vi "LED_test2.vi"() -> ()   [LabVIEW 2012]
uses:
  <vilib>/Utility/file.llb/Read From Spreadsheet File (DBL).vi
  <vilib>/gmath/NI_Gmath.lvlib
  <vilib>/Analysis/NI_AALPro.lvlib
panel:
  out "All Data":string[][](table)
  out "All Counts":dbl[][](array[numeric])
  out "All Abs Irr":dbl[][](array[numeric])
  out "Voltage (Lum)":dbl
  out "Voltage (Cur. Eff.)":dbl
  out "Voltage (EQE)":dbl
  out "Voltage (Lum. Pow. Eff.)":dbl
  in  "Vth_def":dbl=2.1
  out "Von":dbl
  out "Max Cur. Eff.":dbl
  out "Max Lum. Pow. Eff":dbl
  out "Max EQE":dbl
  out "Max Lum.":dbl
  out "Counts/Abs. Irr. vs Wavelength":cluster{"Y":dbl[], "Y":dbl[]}[](graph)
  out "Cur. Eff./Lum. Pow. Eff. vs Voltage":cluster{"Y":dbl[], "Y":dbl[]}[](graph)
  out "Lum. Pow. Eff vs Lum./Cur. Den.":cluster{"Y":dbl[], "Y":dbl[]}[](graph)
  out "Cur. Den. /Lum. vs Voltage":cluster{"Y":dbl[], "Y":dbl[]}[](graph)
  out "Cur. Eff. vs Lum./Cur. Den.":cluster{"Y":dbl[], "Y":dbl[]}[](graph)
  out "x2":dbl=3e-06
  out "x1":dbl=3e-06
  out "WL_1":dbl
  out "WL_2":dbl
  in  "WL_high":dbl=1131.0
  in  "WL_low":dbl=348.0
  out "EQE_array":dbl[](array[numeric])
  out "EQE vs Lum./Cur. Den.":T1(graph)
  out "XY Graph 3":cluster{"Wavelength":dbl[], "Counts":dbl[]}(graph)
  out "Luminance Ratio":dbl[](array[numeric])
  out "Calculated_luminance_array":dbl[](array[numeric])
  out "Calculated_candela_array":dbl[](array[numeric])
  out "Photon_count_array":dbl[](array[numeric])
  out "Photon_count":dbl
  out "Energy_WL":dbl[](array[numeric])
  out "Calculated_candela":dbl
  out "Abs_irr_itpl":dbl[](array[numeric]) format="%_6g"
  out "WL itpl 2":dbl[](array[numeric]) format="%_6g"
  out "Luminous Power Efficiency":dbl[](array[numeric])
  out "current efficiency (Cd/A)":dbl[](array[numeric])
  out "current density (mA/cm2)":dbl[](array[numeric])
  in  "Device Area (m2)":dbl=3e-06
  out "WL_spectrum":dbl[](array[numeric])
  out "Counts_spectrum":dbl[](array[numeric])
  out "Abs_Irr_spectrum":dbl[](array[numeric])
  out "Spectrum":dbl[][](array[numeric])
  out "Counts_dark_spectrum":dbl[](array[numeric])
  out "WL_dark_spectrum":dbl[](array[numeric])
  out "Dark Spectrum all":dbl[][](array[numeric]) format="%0.3f"
  out "Dark_spectrum":dbl[][](array[numeric])
  out "All Spectrum":dbl[][](array[numeric])
  in  "Spectrum File":path=path "W:/LED_quickVIEW/For calibration/20170914_194634spectrum_raw.ciemo"
  out "uW":dbl[](array[numeric])
  out "Luminance":dbl[](array[numeric])
  out "Candela":dbl[](array[numeric])
  out "Current":dbl[](array[numeric])
  out "Voltage":dbl[](array[numeric])
  out "Data":dbl[][](array[numeric]) format="%#.3e"
  in  "Data File":path=path "W:/LED_quickVIEW/For calibration/20170914_194634data.ciemo"
  in  "Calibration File":path=path "W:/LED_quickVIEW/For calibration/2016-12-19 callibration_OOIIrrad.cal_OOIIrrad.cal_OOIIrrad.cal"
  in  "Dark Spectrum File":path=path "W:/LED_quickVIEW/For calibration/20170914_194634dark_reference.ciemo"
  out "max value":dbl
  out "Peak Position":dbl
  out "max index(es)":i32
  out "Iso. Coef. itpl":dbl[](array[numeric]) format="%_6g"
  out "WL itpl":dbl[](array[numeric]) format="%_6g"
  out "XY Graph 2":cluster{"WL":dbl[], "Iso. Coef.":dbl[]}[](graph)
  out "Iso. Coef.":dbl[](array[numeric])
  out "WL":dbl[](array[numeric])
  out "Wavelength":dbl[](array[numeric])
  out "Counts to Abs Irr":dbl[](array[numeric])
  out "XY Graph":cluster{"Wavelength":dbl[], "Counts":dbl[]}(graph)
  out "subarray":dbl[][](array[numeric])
  out "array":dbl[][](array[numeric])
  # "From"
  # "To"
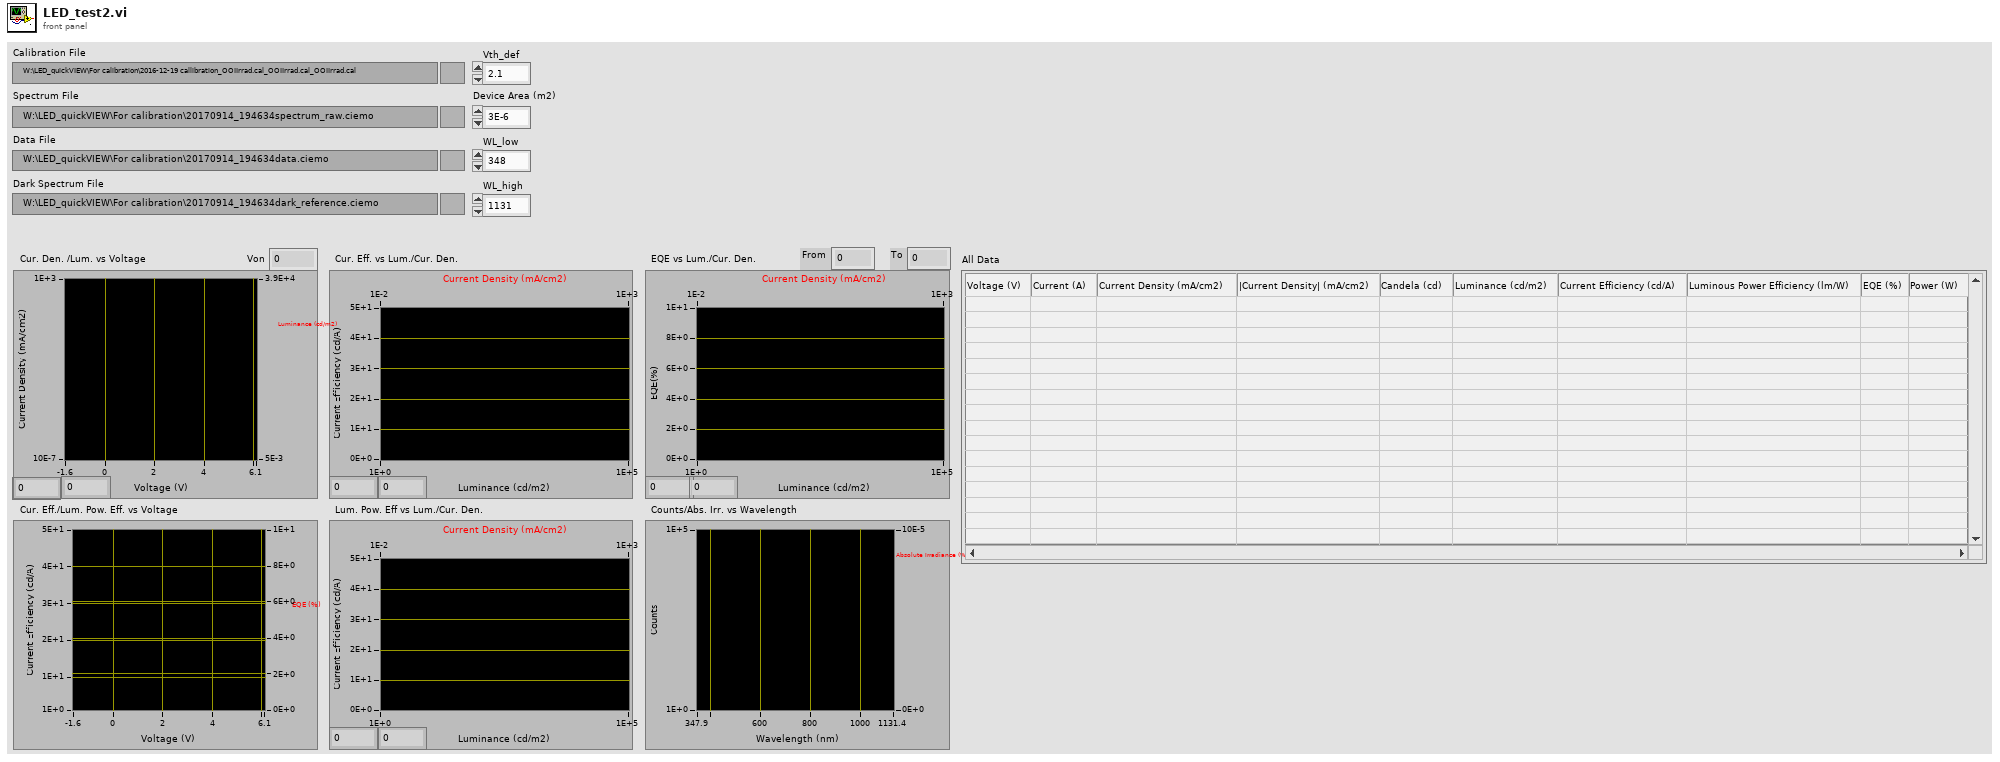
[diagram p1: front panel]
types:
  T1 = cluster{"current density (mA/cm2)":dbl[], "EQE_array":dbl[]}[]
  T2 = cluster{"Wavelength":dbl[], "Counts to Abs Irr":dbl[]}
  T3 = cluster{"WL itpl":dbl[], "Iso. Coef. itpl":dbl[]}
  T4 = cluster{"WL itpl":dbl[], "Iso. Coef. itpl":dbl[]}[]
  T5 = cluster{"Luminance":dbl[], "current efficiency (Cd/A)":dbl[]}
  T6 = cluster{"current density (mA/cm2)":dbl[], "current efficiency (Cd/A)":dbl[]}
  T7 = cluster{"current density (mA/cm2)":dbl[], "EQE_array":dbl[]}
  T8 = cluster{"current density (mA/cm2)":dbl[], "current efficiency (Cd/A)":dbl[]}[]
  T9 = cluster{"Voltage":dbl[], "current efficiency (Cd/A)":dbl[]}
  T10 = cluster{"Luminance":dbl[], "Luminous Power Efficiency":dbl[]}
  T11 = cluster{"current density (mA/cm2)":dbl[], "Luminous Power Efficiency":dbl[]}
  T12 = cluster{"current density (mA/cm2)":dbl[], "Luminous Power Efficiency":dbl[]}[]
  T13 = cluster{"WL_spectrum":dbl[], "Counts_spectrum":dbl[]}
  T14 = cluster{"WL_spectrum":dbl[], "Abs_Irr_spectrum":dbl[]}
  T15 = cluster{"WL_spectrum":dbl[], "Abs_Irr_spectrum":dbl[]}[]
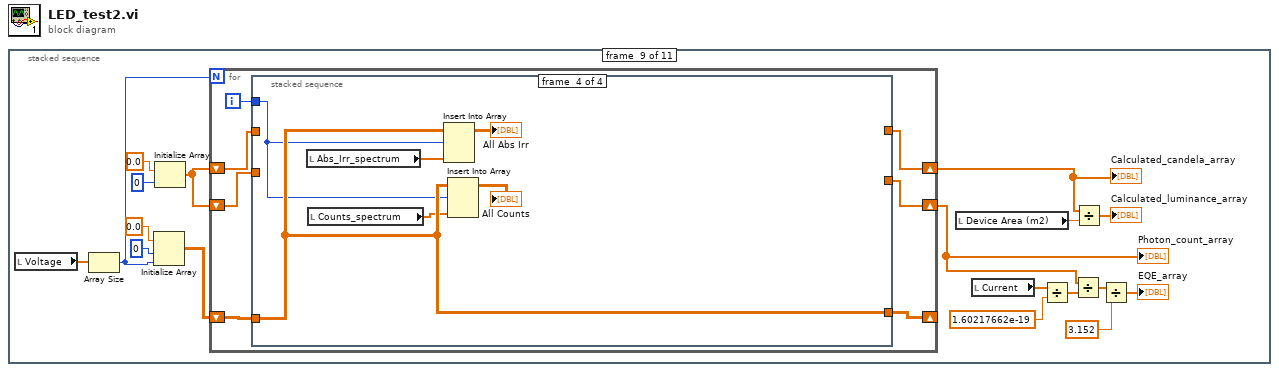
[diagram p0: block diagram]
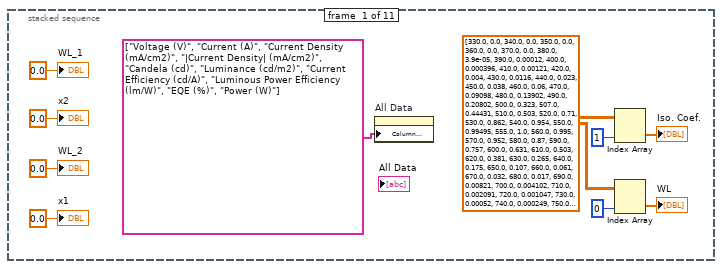
[diagram p2: hidden frame]
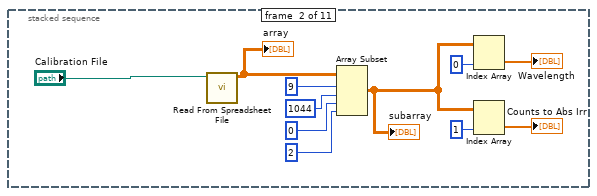
[diagram p3: hidden frame]
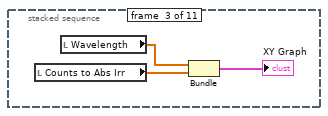
[diagram p4: hidden frame]
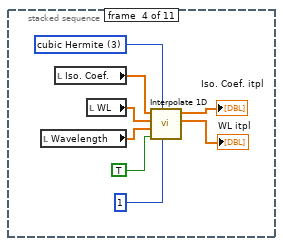
[diagram p5: hidden frame]
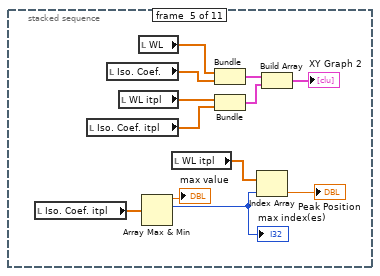
[diagram p6: hidden frame]
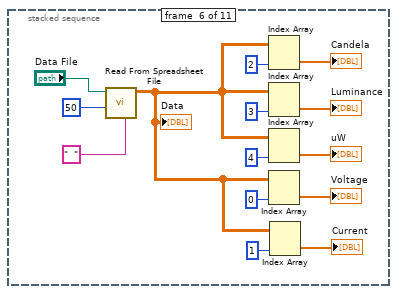
[diagram p7: hidden frame]
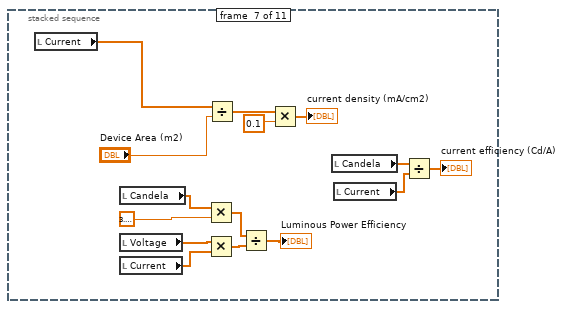
[diagram p8: hidden frame]
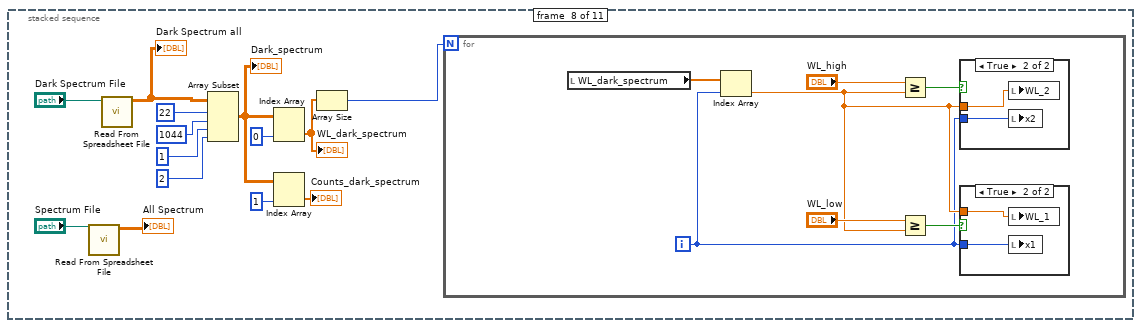
[diagram p9: hidden frame]
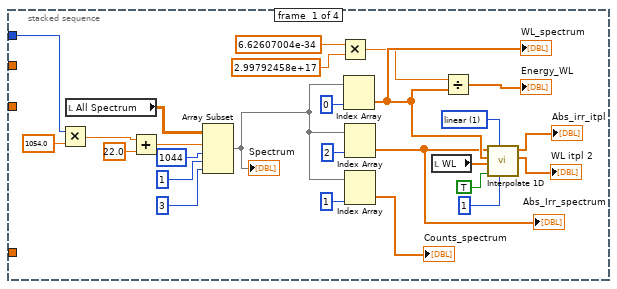
[diagram p12: hidden frame]
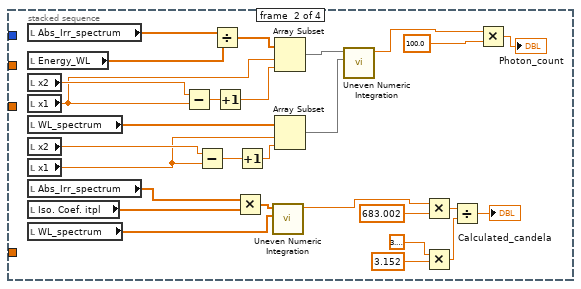
[diagram p13: hidden frame]
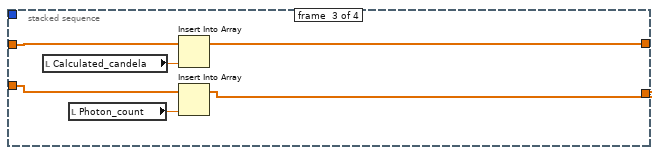
[diagram p14: hidden frame]
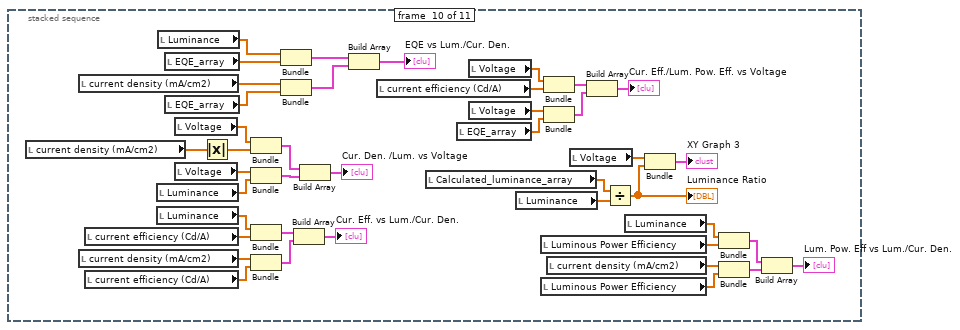
[diagram p15: hidden frame]
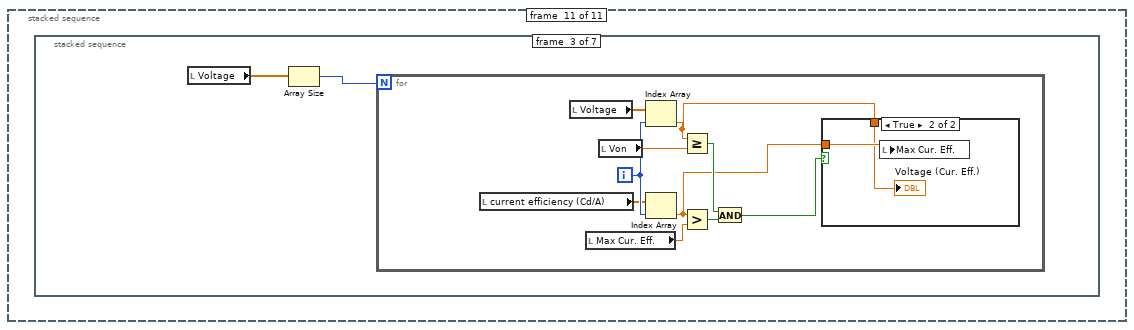
[diagram p16: hidden frame]
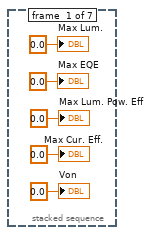
[diagram p17: hidden frame]
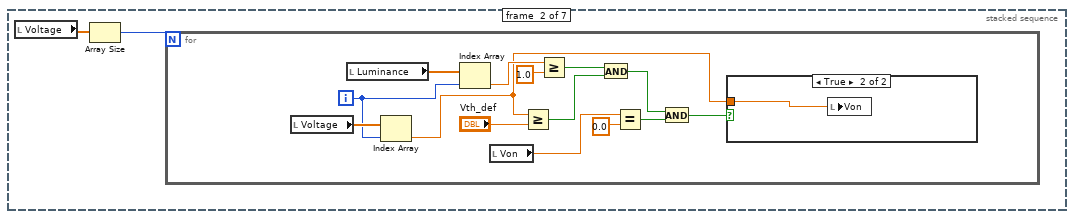
[diagram p18: hidden frame]
diagram:
  n1 = stacked-sequence {
    frame #0 {
      w9 = dbl[][] [[330.0, 0.0], [340.0, 0.0], [350.0, 0.0], [360.0, 0.0], [370.0, 0.0], [380.0, 3.9e-05], [390.0, 0.00012], [400.0, 0.000396], [410.0, 0.00121], [420.0, 0.004], [430.0, 0.0116], [440.0, 0.023], [450.0, 0.038], [460.0, 0.06], [470.0, 0.09098], [480.0, 0.13902], [490.0, 0.20802], [500.0, 0.323], [507.0, 0.44431], [510.0, 0.503], [520.0, 0.71], [530.0, 0.862], [540.0, 0.954], [550.0, 0.99495], [555.0, 1.0], [560.0, 0.995], [570.0, 0.952], [580.0, 0.87], [590.0, 0.757], [600.0, 0.631], [610.0, 0.503], [620.0, 0.381], [630.0, 0.265], [640.0, 0.175], [650.0, 0.107], [660.0, 0.061], [670.0, 0.032], [680.0, 0.017], [690.0, 0.00821], [700.0, 0.004102], [710.0, 0.002091], [720.0, 0.001047], [730.0, 0.00052], [740.0, 0.000249], [750.0, 0.00012], [760.0, 6e-05], [770.0, 3e-05], [780.0, 0.0], [790.0, 0.0], [800.0, 0.0], [810.0, 0.0], [820.0, 0.0], [830.0, 0.0], [840.0, 0.0], [850.0, 0.0], [860.0, 0.0], [870.0, 0.0], [880.0, 0.0], [890.0, 0.0], [900.0, 0.0], [910.0, 0.0], [920.0, 0.0], [930.0, 0.0], [940.0, 0.0], [950.0, 0.0], [960.0, 0.0], [970.0, 0.0], [980.0, 0.0], [990.0, 0.0], [1000.0, 0.0], [1010.0, 0.0], [1020.0, 0.0], [1030.0, 0.0], [1040.0, 0.0], [1050.0, 0.0], [1060.0, 0.0], [1070.0, 0.0], [1080.0, 0.0], [1090.0, 0.0], [1100.0, 0.0], [1110.0, 0.0], [1120.0, 0.0], [1130.0, 0.0], [1140.0, 0.0]] ("all rows")
      n2 = property on="All Data" class="Tbl (strict)"("Column Headers[]"=string[] ["Voltage (V)", "Current (A)", "Current Density (mA/cm2)", "|Current Density| (mA/cm2)", "Candela (cd)", "Luminance (cd/m2)", "Current Efficiency (cd/A)", "Luminous Power Efficiency (lm/W)", "EQE (%)", "Power (W)"] ("Row Header Strings[]")) -> ()  [unwired: 2 in, 2 out]
      n3 = Index Array(array=w9, index (col)=1 ("disabled index (col)")) -> (element=→"Iso. Coef.":dbl[])  [unwired: 1 in]
      n4 = Index Array(array=w9, index (col)=0 ("disabled index (col)")) -> (element=→"WL":dbl[])  [unwired: 1 in]
      "WL_2" <- 0.0 ("WL_2")
      "WL_1" <- 0.0 ("WL_1")
      "x1" <- 0.0 ("x1")
      "x2" <- 0.0 ("x2")
    }
    frame #1 {
      n5 = call-poly <vilib>:"Read From Spreadsheet File.vi"("file path (dialog if empty)"="Calibration File") -> ("all rows"=w18:dbl[][])  [unwired: 6 in, 4 out]
      "array" <- w18
      n6 = Array Subset(array=w18, index (row)=9 ("index"), length (row)=1044 ("length"), index (col)=0 ("index"), length (col)=2 ("length")) -> (w15:dbl[][])
      "subarray" <- w15
      n7 = Index Array(array=w15, index (col)=0 ("index")) -> (element=→"Wavelength":dbl[])  [unwired: 1 in]
      n8 = Index Array(array=w15, index (col)=1 ("length")) -> (element=→"Counts to Abs Irr":dbl[])  [unwired: 1 in]
    }
    frame #2 {
      n9 = local read "Counts to Abs Irr"() -> (w22:dbl[])
      n10 = local read "Wavelength"() -> (w23:dbl[])
      n11 = Bundle("Wavelength"=w23, "Counts to Abs Irr"=w22) -> (→"XY Graph":T2)  [unwired: 1 in]
    }
    frame #3 {
      w28 = 3 items=["nearest", "linear", "spline", "cubic Hermite", "Lagrange"] ("method")
      n12 = local read "Wavelength"() -> (w30:dbl[])
      n13 = local read "Iso. Coef."() -> (w31:dbl[])
      n14 = local read "WL"() -> (w32:dbl[])
      n15 = call <vilib>:"Interpolate 1D.vi"("ntimes"=1, "method"=w28, "X is monotonic"=TRUE, "xi"=w30, "X"=w32, "Y"=w31) -> ("xi used"=→"WL itpl":dbl[], "yi"=→"Iso. Coef. itpl":dbl[])  [unwired: 3 in, 1 out]
    }
    frame #4 {
      n16 = local read "Iso. Coef. itpl"() -> (w37:dbl[])
      n17 = local read "Iso. Coef. itpl"() -> (w33:dbl[])
      n18 = local read "Iso. Coef."() -> (w44:dbl[])
      n19 = local read "WL itpl"() -> (w41:dbl[])
      n20 = local read "WL"() -> (w43:dbl[])
      n21 = Array Max & Min(array=w37) -> (max value=→"max value":dbl, max index (indices)=w40:i32)  [unwired: 2 out]
      "max index(es)" <- w40
      n22 = local read "WL itpl"() -> (w39:dbl[])
      n23 = Bundle("WL"=w43, "Iso. Coef."=w44) -> (w42:cluster{"WL":dbl[], "Iso. Coef.":dbl[]})  [unwired: 1 in]
      n24 = Bundle("WL itpl"=w41, "Iso. Coef. itpl"=w33) -> (w34:T3)  [unwired: 1 in]
      n25 = Index Array(array=w39, index=w40) -> (element=→"Peak Position":dbl)
      n26 = Build Array(w42, w34) -> (→"XY Graph 2":T4)
    }
    frame #5 {
      n27 = call-poly <vilib>:"Read From Spreadsheet File.vi"("delimiter (\\t)"="  " ("delimiter (\\t)"), "start of read offset (chars.:0)"=50, "file path (dialog if empty)"="Data File") -> ("all rows"=w46:dbl[][])  [unwired: 4 in, 4 out]
      "Data" <- w46
      n28 = Index Array(array=w46, index (col)=2 ("index (row)")) -> (element=→"Candela":dbl[])  [unwired: 1 in]
      n29 = Index Array(array=w46, index (col)=3 ("index (row)")) -> (element=→"Luminance":dbl[])  [unwired: 1 in]
      n30 = Index Array(array=w46, index (col)=4 ("index (row)")) -> (element=→"uW":dbl[])  [unwired: 1 in]
      n31 = Index Array(array=w46, index (col)=0 ("index (row)")) -> (element=→"Voltage":dbl[])  [unwired: 1 in]
      n32 = Index Array(array=w46, index (col)=1 ("index (row)")) -> (element=→"Current":dbl[])  [unwired: 1 in]
    }
    frame #6 {
      n33 = local read "Current"() -> (w66:dbl[])
      n34 = local read "Candela"() -> (w61:dbl[])
      n35 = local read "Voltage"() -> (w63:dbl[])
      n36 = local read "Current"() -> (w62:dbl[])
      n37 = Multiply(x=w61, y=3.141592653589793) -> (x*y=w64:dbl[])
      n38 = Multiply(x=w63, y=w62) -> (x*y=w65:dbl[])
      n39 = Divide(x=w66, y="Device Area (m2)") -> (x/y=w71:dbl[])
      n40 = Divide(x=w64, y=w65) -> (x/y=→"Luminous Power Efficiency":dbl[])
      n41 = Multiply(x=w71, y=0.1) -> (x*y=→"current density (mA/cm2)":dbl[])
      n42 = local read "Candela"() -> (w68:dbl[])
      n43 = local read "Current"() -> (w69:dbl[])
      n44 = Divide(x=w68, y=w69) -> (x/y=→"current efficiency (Cd/A)":dbl[])
    }
    frame #7 {
      n45 = call-poly <vilib>:"Read From Spreadsheet File.vi"("file path (dialog if empty)"="Spectrum File") -> ("all rows"=→"All Spectrum":dbl[][])  [unwired: 6 in, 4 out]
      n46 = call-poly <vilib>:"Read From Spreadsheet File.vi"("file path (dialog if empty)"="Dark Spectrum File") -> ("all rows"=w84:dbl[][])  [unwired: 6 in, 4 out]
      "Dark Spectrum all" <- w84
      n47 = Array Subset(array=w84, index (row)=22 ("index"), length (row)=1044 ("length"), index (col)=1 ("index"), length (col)=2 ("length")) -> (w76:dbl[][])
      "Dark_spectrum" <- w76
      n48 = Index Array(array=w76, index (col)=0 ("index")) -> (element=w75:dbl[])  [unwired: 1 in]
      "WL_dark_spectrum" <- w75
      n49 = Index Array(array=w76, index (col)=1 ("index")) -> (element=→"Counts_dark_spectrum":dbl[])  [unwired: 1 in]
      n50 = Array Size(array=w75) -> (size(s)=w74:i32)
      n51 = for {
        N: w74 -> [_]
        i -> [w88]
        n52 = local read "WL_dark_spectrum"() -> (w90:dbl[])
        n53 = Index Array(array=w90, index=w88) -> (element=w89:dbl)
        n54 = Greater Or Equal?(x="WL_high", y=w89) -> (x >= y?=w92:bool)
        n55 = Greater Or Equal?(x="WL_low", y=w89) -> (x >= y?=w91:bool)
        n56 = case shown="True" w92 {
          tunnel: w89 -> [_ w98]
          tunnel: w88 -> [_ w97]
          frame False {
          }
          frame True {
            n57 = local write "WL_2"(w98) -> ()
            n58 = local write "x2"(w97) -> ()
          }
        }
        n59 = case shown="True" w91 {
          tunnel: w89 -> [_ w96]
          tunnel: w88 -> [_ w95]
          frame False {
          }
          frame True {
            n60 = local write "WL_1"(w96) -> ()
            n61 = local write "x1"(w95) -> ()
          }
        }
      }
    }
    frame #8 {
      n62 = local read "Voltage"() -> (w116:dbl[])
      n63 = Array Size(array=w116) -> (size(s)=w101:i32)
      n64 = Initialize Array(0.0 ("element"), 0 ("dimension size"), w101) -> (w99:dbl[][])
      n65 = Initialize Array(0.0 ("element"), 0 ("dimension size")) -> (w103:dbl[])
      n66 = for {
        N: w101 -> [_]
        shift-right: [w121] -> w113
        shift-left: w103 -> [w122]
        shift-right: [w119] -> w108
        shift-left: w103 -> [w120]
        shift-right: [w117] -> _
        shift-left: w99 -> [w118]
        i -> [w123]
        n67 = stacked-sequence {
          tunnel: w123 -> [w137 _ _ w185]
          tunnel: w122 -> [_ _ w182 _]
          tunnel: [_ _ w181 _] -> w121
          tunnel: w120 -> [_ _ w179 _]
          tunnel: [_ _ w178 _] -> w119
          tunnel: w118 -> [_ _ _ w188]
          tunnel: [_ _ _ w188] -> w117
          frame #0 {
            w134 = 1 items=["nearest", "linear", "spline", "cubic Hermite", "Lagrange"] ("method")
            n68 = Multiply(x=w137, y=1054.0) -> (x*y=w147:dbl)
            n69 = local read "All Spectrum"() -> (w136:dbl[][])
            n70 = Add(x=w147, y=22.0) -> (x+y=w149:dbl)
            n71 = Array Subset(array=w136, index (row)=w149, length (row)=1044 ("length"), index (col)=1 ("index"), length (col)=3 ("length")) -> (w140:dbl[][])
            "Spectrum" <- w140
            n72 = Multiply(x=6.62607004e-34, y=2.99792458e+17) -> (x*y=w127:dbl)
            n73 = Index Array(array=w140, index (col)=0 ("index")) -> (element=w131:dbl[])  [unwired: 1 in]
            "WL_spectrum" <- w131
            n74 = Index Array(array=w140, index (col)=2 ("index")) -> (element=w130:dbl[])  [unwired: 1 in]
            "Abs_Irr_spectrum" <- w130
            n75 = Index Array(array=w140, index (col)=1 ("length")) -> (element=→"Counts_spectrum":dbl[])  [unwired: 1 in]
            n76 = local read "WL"() -> (w129:dbl[])
            n77 = Divide(x=w127, y=w131) -> (x/y=→"Energy_WL":dbl[])
            n78 = call <vilib>:"Interpolate 1D.vi"("ntimes"=1, "method"=w134, "X is monotonic"=TRUE, "xi"=w129, "X"=w131, "Y"=w130) -> ("xi used"=→"WL itpl 2":dbl[], "yi"=→"Abs_irr_itpl":dbl[])  [unwired: 3 in, 1 out]
          }
          frame #1 {
            n79 = local read "Abs_Irr_spectrum"() -> (w169:dbl[])
            n80 = local read "Energy_WL"() -> (w168:dbl[])
            n81 = local read "x2"() -> (w155:dbl)
            n82 = local read "x1"() -> (w154:dbl)
            n83 = local read "WL_spectrum"() -> (w151:dbl[])
            n84 = local read "x2"() -> (w153:dbl)
            n85 = local read "x1"() -> (w152:dbl)
            n86 = local read "Abs_Irr_spectrum"() -> (w177:dbl[])
            n87 = local read "Iso. Coef. itpl"() -> (w176:dbl[])
            n88 = local read "WL_spectrum"() -> (w174:dbl[])
            n89 = Subtract(x=w155, y=w154) -> (x-y=w160:dbl)
            n90 = Subtract(x=w153, y=w152) -> (x-y=w157:dbl)
            n91 = Divide(x=w169, y=w168) -> (x/y=w161:dbl[])
            n92 = Increment(x=w160) -> (x+1=w159:dbl)
            n93 = Multiply(x=w177, y=w176) -> (x*y=w175:dbl[])
            n94 = Increment(x=w157) -> (x+1=w156:dbl)
            n95 = call <vilib>:"Uneven Numeric Integration.vi"("T"=w174, "X"=w175) -> ("result"=w172:dbl)  [unwired: 8 in, 1 out]
            n96 = Array Subset(array=w161, index=w154, length=w159) -> (w158:dbl[])
            n97 = Array Subset(array=w151, index=w152, length=w156) -> (w150:dbl[])
            n98 = call <vilib>:"Uneven Numeric Integration.vi"("T"=w150, "X"=w158) -> ("result"=w167:dbl)  [unwired: 8 in, 1 out]
            n99 = Multiply(x=w172, y=683.002) -> (x*y=w173:dbl)
            n100 = Multiply(x=3.141592653589793, y=3.152) -> (x*y=w163:dbl)
            n101 = Divide(x=w173, y=w163) -> (x/y=→"Calculated_candela":dbl)
            n102 = Multiply(x=w167, y=100.0) -> (x*y=→"Photon_count":dbl)
          }
          frame #2 {
            n103 = local read "Calculated_candela"() -> (w183:dbl)
            n104 = local read "Photon_count"() -> (w180:dbl)
            n105 = Insert Into Array(array=w182, new element=w183) -> (w181:dbl[])  [unwired: 1 in]
            n106 = Insert Into Array(array=w179, new element=w180) -> (w178:dbl[])  [unwired: 1 in]
          }
          frame #3 {
            n107 = local read "Abs_Irr_spectrum"() -> (w189:dbl[])
            n108 = local read "Counts_spectrum"() -> (w187:dbl[])
            n109 = Insert Into Array(array=w188, index (row)=w185, new element=w189) -> (→"All Abs Irr":dbl[][])  [unwired: 1 in]
            n110 = Insert Into Array(array=w188, index (row)=w185, new element=w187) -> (→"All Counts":dbl[][])  [unwired: 1 in]
          }
        }
      }
      "Photon_count_array" <- w108
      "Calculated_candela_array" <- w113
      n111 = local read "Device Area (m2)"() -> (w111:dbl)
      n112 = local read "Current"() -> (w110:dbl[])
      n113 = Divide(x=w110, y=1.60217662e-19) -> (x/y=w109:dbl[])
      n114 = Divide(x=w108, y=w109) -> (x/y=w106:dbl[])
      n115 = Divide(x=w113, y=w111) -> (x/y=→"Calculated_luminance_array":dbl[])
      n116 = Divide(x=w106, y=3.152) -> (x/y=→"EQE_array":dbl[])
    }
    frame #9 {
      n117 = local read "current density (mA/cm2)"() -> (w212:dbl[])
      n118 = local read "current density (mA/cm2)"() -> (w222:dbl[])
      n119 = local read "current density (mA/cm2)"() -> (w205:dbl[])
      n120 = local read "current efficiency (Cd/A)"() -> (w207:dbl[])
      n121 = local read "current efficiency (Cd/A)"() -> (w204:dbl[])
      n122 = local read "Luminance"() -> (w213:dbl[])
      n123 = local read "Luminance"() -> (w206:dbl[])
      n124 = local read "Luminance"() -> (w223:dbl[])
      n125 = local read "EQE_array"() -> (w224:dbl[])
      n126 = local read "EQE_array"() -> (w225:dbl[])
      n127 = local read "Voltage"() -> (w215:dbl[])
      n128 = local read "Voltage"() -> (w214:dbl[])
      n129 = Absolute Value(x=w212) -> (abs(x)=w211:dbl[])
      n130 = Bundle("Voltage"=w215, w211) -> (w218:cluster{"Voltage":dbl[], dbl[]})  [unwired: 1 in]
      n131 = Bundle("Voltage"=w214, "Luminance"=w213) -> (w217:cluster{"Voltage":dbl[], "Luminance":dbl[]})  [unwired: 1 in]
      n132 = Bundle("Luminance"=w206, "current efficiency (Cd/A)"=w207) -> (w210:T5)  [unwired: 1 in]
      n133 = Bundle("current density (mA/cm2)"=w205, "current efficiency (Cd/A)"=w204) -> (w209:T6)  [unwired: 1 in]
      n134 = Bundle("Luminance"=w223, "EQE_array"=w224) -> (w221:cluster{"Luminance":dbl[], "EQE_array":dbl[]})  [unwired: 1 in]
      n135 = Bundle("current density (mA/cm2)"=w222, "EQE_array"=w225) -> (w220:T7)  [unwired: 1 in]
      n136 = Build Array(w210, w209) -> (→"Cur. Eff. vs Lum./Cur. Den.":T8)
      n137 = Build Array(w218, w217) -> (→"Cur. Den. /Lum. vs Voltage":cluster{"Voltage":dbl[], "Luminance":dbl[]}[])
      n138 = Build Array(w221, w220) -> (→"EQE vs Lum./Cur. Den.":T1)
      n139 = local read "current efficiency (Cd/A)"() -> (w191:dbl[])
      n140 = local read "Calculated_luminance_array"() -> (w229:dbl[])
      n141 = local read "EQE_array"() -> (w190:dbl[])
      n142 = local read "Voltage"() -> (w193:dbl[])
      n143 = local read "Voltage"() -> (w192:dbl[])
      n144 = local read "Luminance"() -> (w230:dbl[])
      n145 = local read "Luminous Power Efficiency"() -> (w199:dbl[])
      n146 = local read "Luminous Power Efficiency"() -> (w197:dbl[])
      n147 = Bundle("Voltage"=w193, "current efficiency (Cd/A)"=w191) -> (w196:T9)  [unwired: 1 in]
      n148 = Bundle("Voltage"=w192, "EQE_array"=w190) -> (w195:cluster{"Voltage":dbl[], "EQE_array":dbl[]})  [unwired: 1 in]
      n149 = local read "current density (mA/cm2)"() -> (w198:dbl[])
      n150 = local read "Voltage"() -> (w228:dbl[])
      n151 = Build Array(w196, w195) -> (→"Cur. Eff./Lum. Pow. Eff. vs Voltage":cluster{"Voltage":dbl[], "EQE_array":dbl[]}[])
      n152 = Divide(x=w229, y=w230) -> (x/y=w227:dbl[])
      "Luminance Ratio" <- w227
      n153 = local read "Luminance"() -> (w200:dbl[])
      n154 = Bundle("Voltage"=w228, w227) -> (→"XY Graph 3":cluster{"Voltage":dbl[], dbl[]})  [unwired: 1 in]
      n155 = Bundle("Luminance"=w200, "Luminous Power Efficiency"=w199) -> (w203:T10)  [unwired: 1 in]
      n156 = Bundle("current density (mA/cm2)"=w198, "Luminous Power Efficiency"=w197) -> (w202:T11)  [unwired: 1 in]
      n157 = Build Array(w203, w202) -> (→"Lum. Pow. Eff vs Lum./Cur. Den.":T12)
    }
    frame #10 {
      n158 = stacked-sequence {
        frame #0 {
          "Max Lum." <- 0.0 ("element")
          "Max EQE" <- 0.0 ("element")
          "Max Lum. Pow. Eff" <- 0.0 ("element")
          "Max Cur. Eff." <- 0.0 ("element")
          "Von" <- 0.0 ("element")
        }
        frame #1 {
          n159 = local read "Voltage"() -> (w236:dbl[])
          n160 = Array Size(array=w236) -> (size(s)=w237:i32)
          n161 = for {
            N: w237 -> [_]
            i -> [w247]
            n162 = local read "Voltage"() -> (w249:dbl[])
            n163 = local read "Luminance"() -> (w248:dbl[])
            n164 = Index Array(array=w249, index=w247) -> (element=w238:dbl)
            n165 = Index Array(array=w248, index=w247) -> (element=w246:dbl)
            n166 = local read "Von"() -> (w243:dbl)
            n167 = Greater Or Equal?(x=w238, y="Vth_def") -> (x >= y?=w251:bool)
            n168 = Greater Or Equal?(x=w246, y=1.0) -> (x >= y?=w244:bool)
            n169 = And(x=w244, y=w251) -> (x .and. y?=w240:bool)
            n170 = Equal?(x=w243, y=0.0) -> (x = y?=w241:bool)
            n171 = And(x=w240, y=w241) -> (x .and. y?=w239:bool)
            n172 = case shown="True" w239 {
              tunnel: w238 -> [_ w252]
              frame False {
              }
              frame True {
                n173 = local write "Von"(w252) -> ()
              }
            }
          }
        }
        frame #2 {
          n174 = local read "Voltage"() -> (w253:dbl[])
          n175 = Array Size(array=w253) -> (size(s)=w254:i32)
          n176 = for {
            N: w254 -> [_]
            i -> [w260]
            n177 = local read "current efficiency (Cd/A)"() -> (w259:dbl[])
            n178 = local read "Voltage"() -> (w264:dbl[])
            n179 = local read "Max Cur. Eff."() -> (w261:dbl)
            n180 = local read "Von"() -> (w263:dbl)
            n181 = Index Array(array=w264, index=w260) -> (element=w255:dbl)
            n182 = Index Array(array=w259, index=w260) -> (element=w256:dbl)
            n183 = Greater Or Equal?(x=w255, y=w263) -> (x >= y?=w262:bool)
            n184 = Greater?(x=w256, y=w261) -> (0:w258:bool)
            n185 = And(x=w262, y=w258) -> (x .and. y?=w257:bool)
            n186 = case shown="True" w257 {
              tunnel: w256 -> [_ w266]
              tunnel: w255 -> [_ w265]
              frame False {
              }
              frame True {
                n187 = local write "Max Cur. Eff."(w266) -> ()
                "Voltage (Cur. Eff.)" <- w265
              }
            }
          }
        }
        frame #3 {
          n188 = local read "Voltage"() -> (w267:dbl[])
          n189 = Array Size(array=w267) -> (size(s)=w268:i32)
          n190 = for {
            N: w268 -> [_]
            i -> [w274]
            n191 = local read "EQE_array"() -> (w273:dbl[])
            n192 = local read "Voltage"() -> (w278:dbl[])
            n193 = local read "Von"() -> (w277:dbl)
            n194 = local read "Max EQE"() -> (w275:dbl)
            n195 = Index Array(array=w278, index=w274) -> (element=w269:dbl)
            n196 = Index Array(array=w273, index=w274) -> (element=w270:dbl)
            n197 = Greater Or Equal?(x=w269, y=w277) -> (x >= y?=w276:bool)
            n198 = Greater?(x=w270, y=w275) -> (0:w272:bool)
            n199 = And(x=w276, y=w272) -> (x .and. y?=w271:bool)
            n200 = case shown="True" w271 {
              tunnel: w270 -> [_ w280]
              tunnel: w269 -> [_ w279]
              frame False {
              }
              frame True {
                n201 = local write "Max EQE"(w280) -> ()
                "Voltage (EQE)" <- w279
              }
            }
          }
        }
        frame #4 {
          n202 = local read "Voltage"() -> (w281:dbl[])
          n203 = Array Size(array=w281) -> (size(s)=w282:i32)
          n204 = for {
            N: w282 -> [_]
            i -> [w288]
            n205 = local read "Luminous Power Efficiency"() -> (w287:dbl[])
            n206 = local read "Max Lum. Pow. Eff"() -> (w289:dbl)
            n207 = local read "Voltage"() -> (w292:dbl[])
            n208 = local read "Von"() -> (w291:dbl)
            n209 = Index Array(array=w292, index=w288) -> (element=w283:dbl)
            n210 = Index Array(array=w287, index=w288) -> (element=w284:dbl)
            n211 = Greater Or Equal?(x=w283, y=w291) -> (x >= y?=w290:bool)
            n212 = Greater?(x=w284, y=w289) -> (0:w286:bool)
            n213 = And(x=w290, y=w286) -> (x .and. y?=w285:bool)
            n214 = case shown="True" w285 {
              tunnel: w284 -> [_ w294]
              tunnel: w283 -> [_ w293]
              frame False {
              }
              frame True {
                n215 = local write "Max Lum. Pow. Eff"(w294) -> ()
                "Voltage (Lum. Pow. Eff.)" <- w293
              }
            }
          }
        }
        frame #5 {
          n216 = local read "Voltage"() -> (w295:dbl[])
          n217 = Array Size(array=w295) -> (size(s)=w296:i32)
          n218 = for {
            N: w296 -> [_]
            i -> [w302]
            n219 = local read "Luminance"() -> (w301:dbl[])
            n220 = local read "Voltage"() -> (w306:dbl[])
            n221 = local read "Von"() -> (w305:dbl)
            n222 = local read "Max Lum."() -> (w303:dbl)
            n223 = Index Array(array=w306, index=w302) -> (element=w297:dbl)
            n224 = Index Array(array=w301, index=w302) -> (element=w298:dbl)
            n225 = Greater Or Equal?(x=w297, y=w305) -> (x >= y?=w304:bool)
            n226 = Greater?(x=w298, y=w303) -> (0:w300:bool)
            n227 = And(x=w304, y=w300) -> (x .and. y?=w299:bool)
            n228 = case shown="True" w299 {
              tunnel: w298 -> [_ w308]
              tunnel: w297 -> [_ w307]
              frame False {
              }
              frame True {
                n229 = local write "Max Lum."(w308) -> ()
                "Voltage (Lum)" <- w307
              }
            }
          }
        }
        frame #6 {
          n230 = local read "Counts_spectrum"() -> (w310:dbl[])
          n231 = local read "Abs_Irr_spectrum"() -> (w309:dbl[])
          n232 = local read "WL_spectrum"() -> (w311:dbl[])
          n233 = local read "WL_spectrum"() -> (w312:dbl[])
          n234 = Bundle("WL_spectrum"=w311, "Counts_spectrum"=w310) -> (w315:T13)  [unwired: 1 in]
          n235 = Bundle("WL_spectrum"=w312, "Abs_Irr_spectrum"=w309) -> (w314:T14)  [unwired: 1 in]
          n236 = Build Array(w315, w314) -> (→"Counts/Abs. Irr. vs Wavelength":T15)
        }
      }
    }
  }
